vi "SetAdGain_thread.vi"(1 "gain":u8=6, 2 "board":u32) -> ()   [LabVIEW 2015]
uses:
  lv64_eventdriven/board.vis/ESLSCDLL.dll
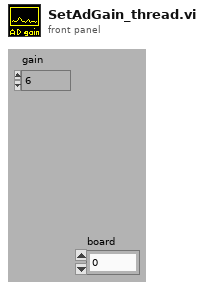
[diagram p1: front panel]
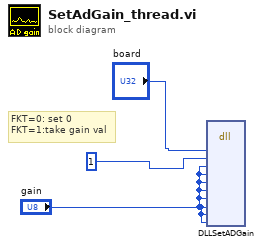
[diagram p0: block diagram]
diagram:
  # "FKT=0: set 0\nFKT=1:take gain val"
  n1 = dll-call lib="C:/ENTW/PCIE/64bit/lv64/lv64_eventdriven/board.vis/ESLSCDLL.dll" fn="DLLSetADGain" ("lwlscdll.dll:DLLSetADAmpRed")("drv"="board", "fkt"=u8 1, "g1"="gain", "g2"="gain", "g3"="gain", "g4"="gain", "g5"="gain", "g6"="gain", "g7"="gain", "g8"="gain") -> ()  [unwired: 14 in, 2 out]
